vi "Init.vi"(8 "error in (no error)":errorcluster, 11 "HighscoreDialog in":refnum<class "HighscoreDialog.lvclass">) -> (0 "error out":errorcluster, 3 "HighscoreDialog out":refnum<class "HighscoreDialog.lvclass">)   [LabVIEW 2019, in "RT_Game.lvlib" / "HighscoreDialog.lvclass"]
uses:
  HighscoreDialog.lvclass
  HighscoreDialog.lvclass/HighscoreDialog.ctl
  GameObject/GameObject.lvclass
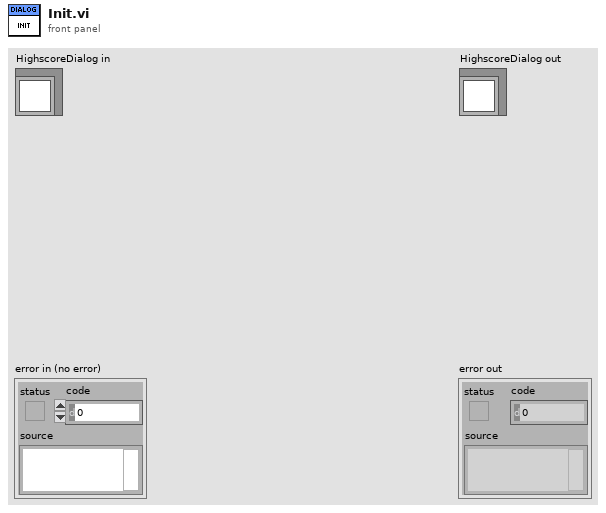
[diagram p1: front panel]
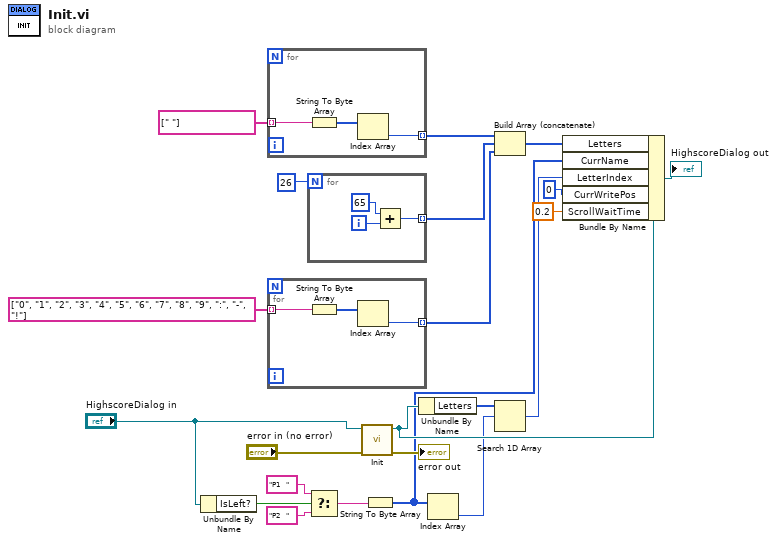
[diagram p0: block diagram]
diagram:
  n1 = Unbundle By Name("HighscoreDialog in") -> ("IsLeft?"=w10:bool)
  n2 = for {
    tunnel: string[] [" "] ("GameName") -> [w25] mode=indexing
    tunnel: [w23] -> w19 mode=indexing
    n3 = String To Byte Array(string=w25) -> (unsigned byte array=w24:u8[])
    n4 = Index Array(array=w24) -> (element=w23:u8)  [unwired: 1 in]
  }
  n5 = for {
    tunnel: string[] ["0", "1", "2", "3", "4", "5", "6", "7", "8", "9", ":", "-", "!"] ("GameName") -> [w28] mode=indexing
    tunnel: [w26] -> w17 mode=indexing
    n6 = String To Byte Array(string=w28) -> (unsigned byte array=w27:u8[])
    n7 = Index Array(array=w27) -> (element=w26:u8)  [unwired: 1 in]
  }
  n8 = for {
    N: 26 -> [_]
    tunnel: [w29] -> w15 mode=indexing
    i -> [w30]
    n9 = Add(x=65 ("Numeric"), y=w30) -> (x+y=w29:i32)
  }
  n10 = Select(t="P1   " ("GameName"), s=w10, f="P2   " ("GameName")) -> (s? t:f=w8:string)
  n11 = call-parent "Init.vi"("error in (no error)"="error in (no error)", "GameObject in"="HighscoreDialog in") -> ("error out"=→"error out":errorcluster, "GameObject out"=w7:refnum<class "HighscoreDialog.lvclass">)  [unwired: 8 in]
  n12 = String To Byte Array(string=w8) -> (unsigned byte array=w4:u8[])
  n13 = Unbundle By Name(w7) -> ("Letters"=w6:u8[])
  n14 = Index Array(array=w4) -> (element=w3:u8)  [unwired: 1 in]
  n15 = Build Array (concatenate)(w19, w15, w17) -> (w14:i32[])
  n16 = Search 1D Array(1D array=w6, element=w3) -> (index of element=w2:i32)  [unwired: 1 in]
  n17 = Bundle By Name(cluster=w7, "Letters"=w14, "CurrName"=w4, "LetterIndex"=w2, "CurrWritePos"=i16 0, "ScrollWaitTime"=0.2) -> (→"HighscoreDialog out":refnum<class "HighscoreDialog.lvclass">)
